vi "WT1600 Integrator Query.vi"(8 "error in (no error)":errorcluster, 9 "Element":u32=1 min=1 step=1, 11 "VISA resource name":refnum<visa-resource-name>) -> (0 "error out":errorcluster, 1 "Response":string, 3 "VISA resource name out":refnum<visa-resource-name>)   [LabVIEW 2012, in "WT1600.lvlib"]
doc: "This VI query the Yokogawa WT1600 for the integration state of the specified element. The possibile returns are:\n\nRES for reset\nSTAR for start\nSTOP for stop"
uses:
  Generic Instrument/WT1600 Card/WT1600/WT1600.lvlib
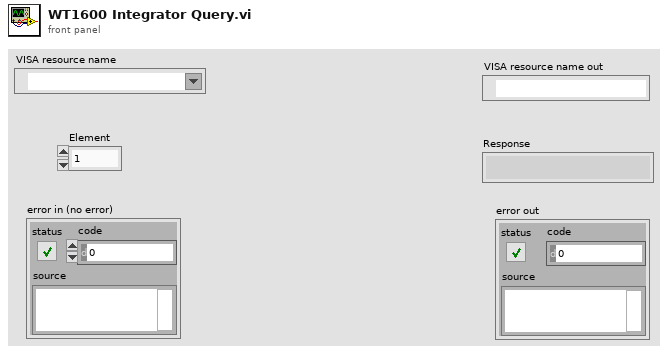
[diagram p1: front panel]
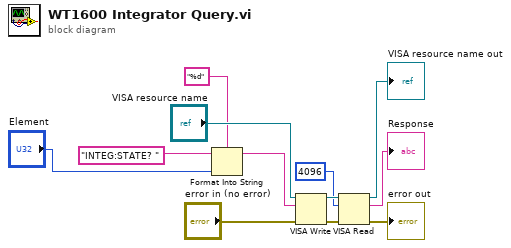
[diagram p0: block diagram]
diagram:
  n1 = Format Into String(format string="%d", initial string="INTEG:STATE? " ("write buffer"), "Element") -> (resulting string=w2:string)  [unwired: 1 in, 1 out]
  n2 = VISA Write(VISA resource name="VISA resource name", write buffer=w2, error in (no error)="error in (no error)") -> (VISA resource name out=w12:refnum<visa-resource-name>, error out=w11:errorcluster)  [unwired: 1 out]
  n3 = VISA Read(VISA resource name=w12, byte count=u32 4096, error in (no error)=w11) -> (VISA resource name out=→"VISA resource name out":refnum<visa-resource-name>, read buffer=→"Response":string, error out=→"error out":errorcluster)  [unwired: 1 out]
